vi "TCP_IP Jayasingha Richou Odier.vi"() -> ()   [LabVIEW 2019]
panel:
  out "VIBRATION ANGLE":dynamicdata(graph)
  out "VOL  DB":dynamicdata(graph)
  out "GAZ PPM":dynamicdata(graph)
  out "LUMINOSITE LUX":dynamicdata(graph)
  out "HUMIDITE %":dynamicdata(graph)
  out "TEMPERATURE":dynamicdata(graph)
  out "Nombre de lignes lues":i32
  out "?":dbl
  out "?":dbl
  out "?":dbl
  out "?":dbl
  out "CUMUL DES POINTS":dbl
  out "Oui (vert) / Non (rouge)":bool
  out "Points gaz":dbl
  out "Points Humidité":dbl
  out "Points Temperature":dbl
  out "?":dbl(slide) scale=0.0..0.005
  out "?":dbl(slide) scale=0.0..0.005
  out "?":dbl(slide) scale=0.0..0.005
  out "?":dbl(slide) scale=0.0..0.005
  out "?":dbl(slide) scale=0.0..0.005
  out "?":dbl(slide) scale=0.0..0.005
  out "?":dbl(slide) scale=0.0..0.005
  out "Données de sortie":dbl[][](array[numeric])
  out "Valeur de la  i ème ligne lue":dbl[](array[numeric])
  in  "stop":bool
  # "COUNTER"
  # "HUMIDITÉ"
  # "TEMPERATURE"
  # "LUMINOSITÉ"
  # "GAZ"
  # "VOLUME PIC"
  # "VOLUME AMBIANT"
  # "VIBRATIONS"
  # "A t il le droit d'avoir une compensation ?"
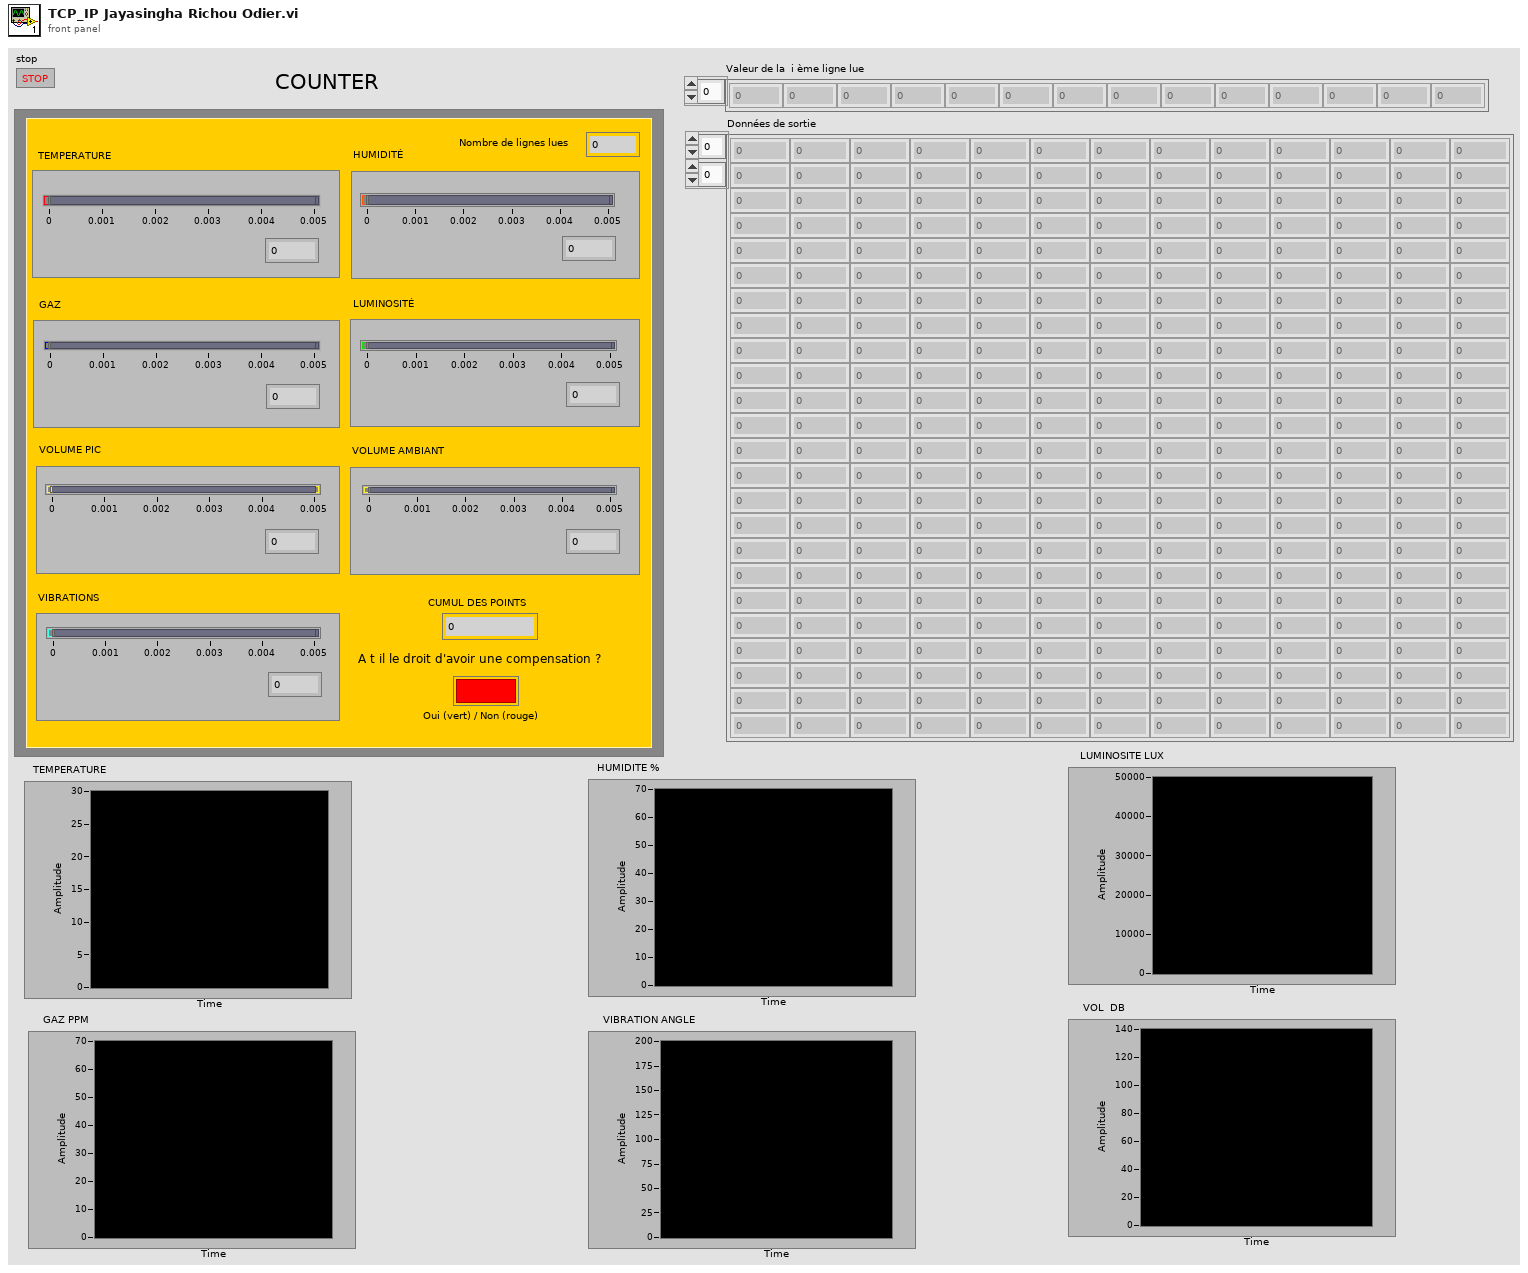
[diagram p1: front panel]
types:
  T1 = enum16{"Standard", "Buffered", "CRLF", "Immediate"}
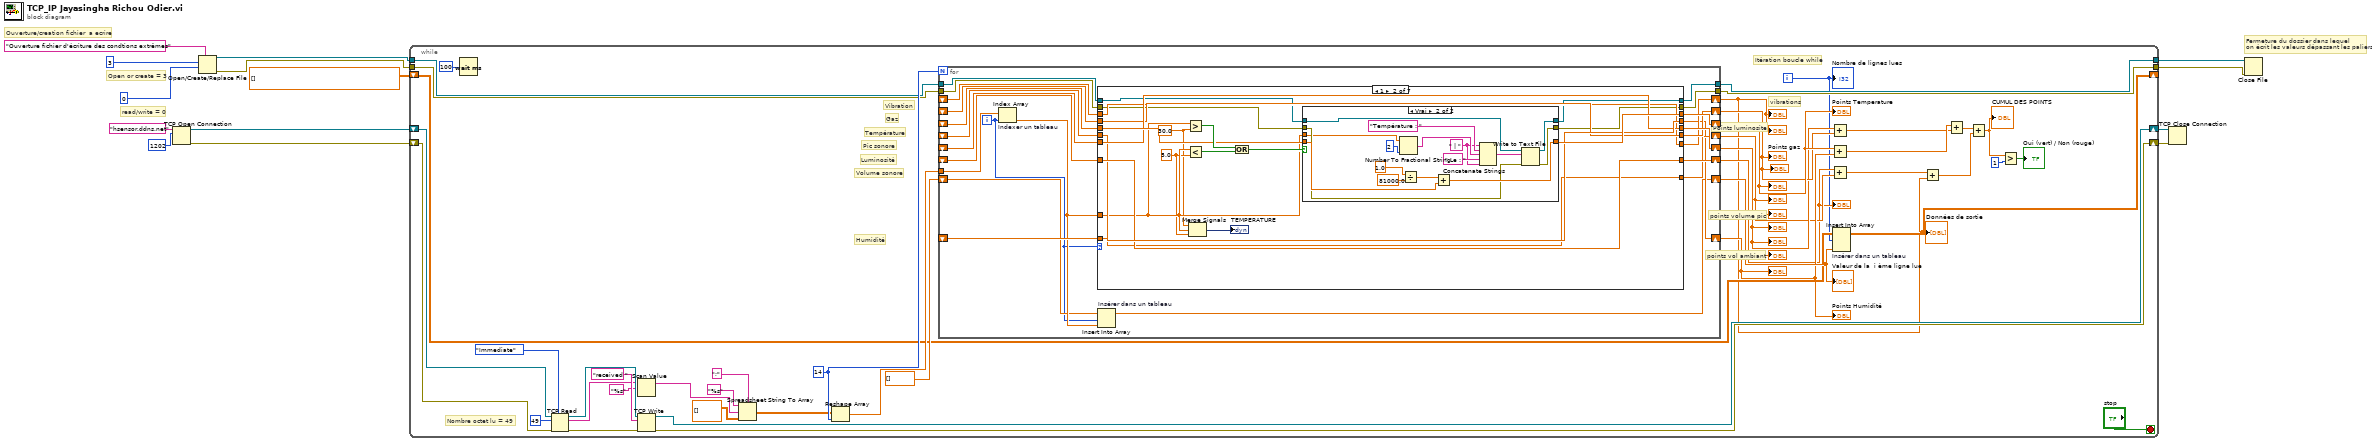
[diagram p0: block diagram]
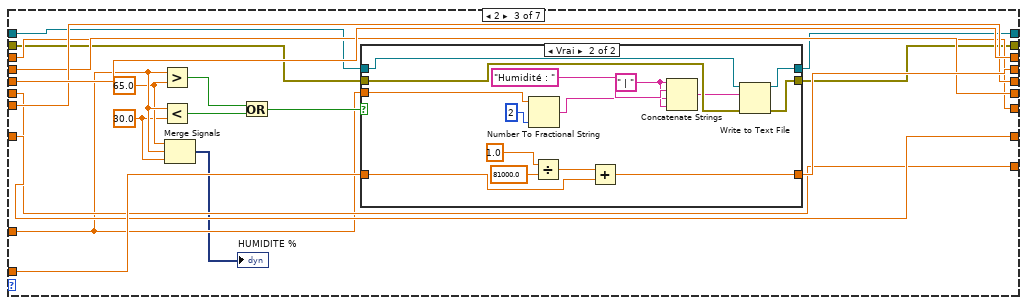
[diagram p4: hidden frame]
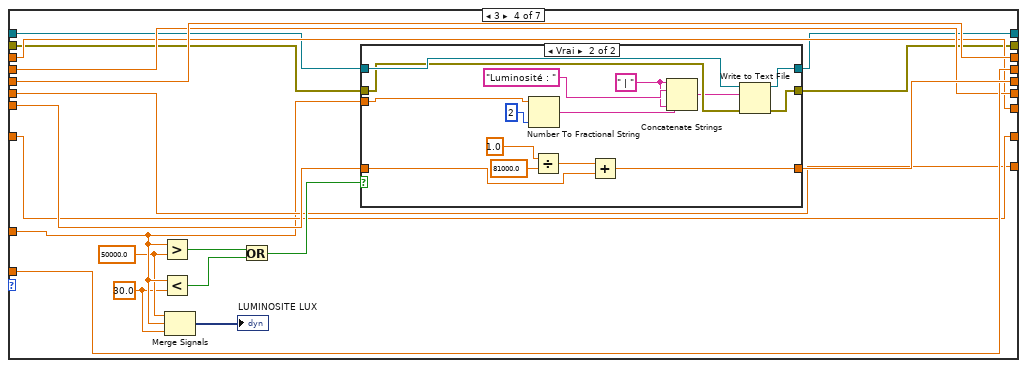
[diagram p6: hidden frame]
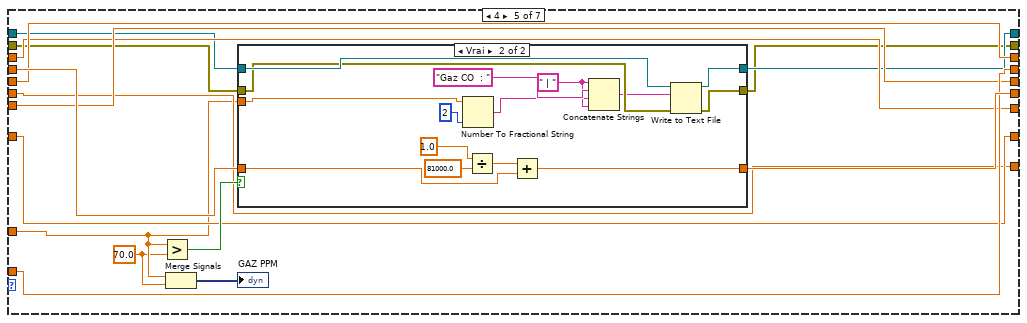
[diagram p8: hidden frame]
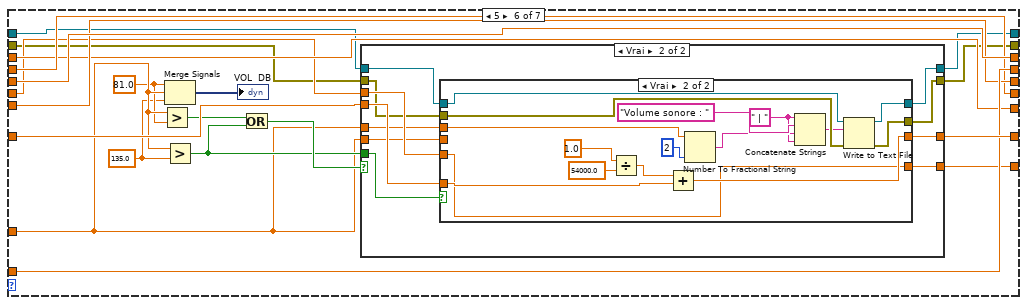
[diagram p10: hidden frame]
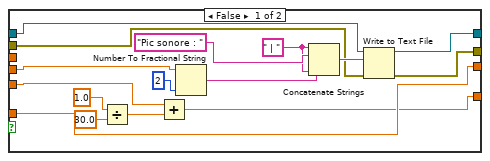
[diagram p12: hidden frame]
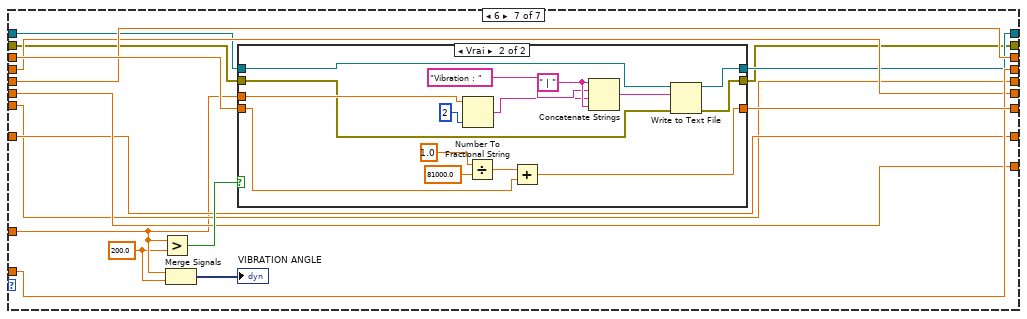
[diagram p13: hidden frame]
diagram:
  # "Fermeture du dossier dans lequel \non écrit les valeurs dépassant les paliers"
  # "read/write = 0"
  # "Open or create = 3"
  # "Ouverture/creation fichier  a ecrire"
  n1 = TCP Open Connection(address="hsensor.ddns.net", remote port or service name=u16 1202) -> (connection ID=w10:refnum<k5>, error out=w9:errorcluster)  [unwired: 3 in]
  n2 = Open/Create/Replace File(prompt="Ouverture fichier d'écriture des condtions extrêmes", operation (0:open)=3, access (0:read/write)=0) -> (refnum out=w3:refnum<file>, error out=w4:errorcluster)  [unwired: 3 in, 1 out]
  n3 = while {
    shift-right: [w57] -> w14
    shift-left: w9 -> [w55]
    shift-right: [w53] -> w11
    shift-left: w10 -> [w52]
    shift-right: [w27] -> _
    shift-left: dbl[][] [] ("array type (2D Dbl)") -> [w29]
    tunnel: w4 -> [w26]
    tunnel: w3 -> [w25]
    tunnel: [w24] -> w2
    tunnel: [w23] -> w1
    i -> [w15]
    stop <- "stop" stop-if-true
    w42 = 14 ("dimension size")
    # "Itération boucle while"
    # "vibrations"
    # "points vol ambiant"
    # "points volume pic"
    # "Points luminosite"
    # "Nombre octet lu = 49"
    # "Vibration"
    # "Pic sonore"
    # "Volume sonore"
    # "Gaz"
    # "Luminosité"
    # "Humidité"
    # "Température"
    n4 = Wait (ms)(milliseconds to wait=u32 100) -> ()  [unwired: 1 out]
    n5 = TCP Read(connection ID=w52, bytes to read=49, error in (no error)=w55, 7:T1."Immediate" ("mode (standard)")) -> (connection ID out=w54:refnum<k5>, data out=w47:string, error out=w58:errorcluster)  [unwired: 1 in]
    n6 = Scan Value(string=w47, format string="%s") -> (output string=w32:string)  [unwired: 1 in, 1 out]
    n7 = TCP Write(connection ID=w54, data in="received " ("data out"), error in (no error)=w58) -> (connection ID out=w53:refnum<k5>, error out=w57:errorcluster)  [unwired: 1 in, 1 out]
    n8 = Spreadsheet String To Array(delimiter (Tab)=";", format string="%s", spreadsheet string=w32, array type (2D Dbl)=dbl[][] []) -> (array=w28:dbl[][])
    n9 = Reshape Array "Reshape Array"(w28, w42) -> (w41:dbl[])
    n10 = for {
      N: w42 -> [_]
      shift-right: [w65] -> w30
      shift-left: dbl[] [] ("array type (2D Dbl)") -> [w66]
      tunnel: w41 -> [w59]
      shift-right: [w81] -> w22
      shift-left: _ -> [w80]
      shift-right: [w69] -> w21
      shift-left: _ -> [w68]
      shift-right: [w78] -> w19
      shift-left: _ -> [w79]
      shift-right: [w76] -> w20
      shift-left: _ -> [w77]
      shift-right: [w74] -> w17
      shift-left: _ -> [w75]
      shift-right: [w72] -> w18
      shift-left: _ -> [w73]
      shift-right: [w71] -> w16
      shift-left: _ -> [w70]
      tunnel: w26 -> [w64]
      tunnel: w25 -> [w63]
      tunnel: [w62] -> w24
      tunnel: [w61] -> w23
      i -> [w60]
      n11 = Index Array "Indexer un tableau"(array=w59, index=w60) -> (element=w67:dbl)
      n12 = case shown="1" w60 {
        tunnel: [w90 w106 w142 w179 w215 w254 w316] -> w81
        tunnel: w80 -> [w90 w105 w142 w179 w215 w254 w316]
        tunnel: [w89 w104 w144 w178 w214 w253 w315] -> w69
        tunnel: w79 -> [w88 w103 w141 w180 w213 w252 w311]
        tunnel: [w88 w103 w141 w181 w213 w252 w311] -> w78
        tunnel: w77 -> [w87 w102 w140 w177 w218 w251 w312]
        tunnel: [w87 w102 w140 w177 w216 w251 w312] -> w76
        tunnel: w75 -> [w86 w101 w139 w176 w212 w256 w313]
        tunnel: [w86 w101 w139 w176 w212 w255 w313] -> w74
        tunnel: w73 -> [w85 w100 w138 w175 w211 w246 w314]
        tunnel: [w85 w100 w138 w175 w211 w245 w314] -> w72
        tunnel: [w84 w99 w137 w174 w210 w250 w318] -> w71
        tunnel: w70 -> [w84 w99 w137 w174 w210 w250 w317]
        tunnel: w68 -> [w89 w104 w143 w178 w214 w253 w315]
        tunnel: w67 -> [_ w94 w132 w169 w205 w240 w306]
        tunnel: w64 -> [w83 w98 w135 w172 w208 w243 w310]
        tunnel: w63 -> [w82 w97 w136 w173 w209 w244 w309]
        tunnel: [w83 w96 w134 w171 w206 w241 w307] -> w62
        tunnel: [w82 w95 w133 w170 w207 w242 w308] -> w61
        frame 0, Default {
        }
        frame 1 {
          w93 = 5.0 ("y")
          w92 = 30.0 ("y")
          n13 = Greater?(x=w94, y=w92) -> (0:w109:bool)
          n14 = Less?(x=w94, y=w93) -> (x < y?=w108:bool)
          n15 = Merge Signals(w92, w94, w93) -> (→"TEMPERATURE":dynamicdata)
          n16 = Or(x=w109, y=w108) -> (x .or. y?=w107:bool)
          n17 = case shown="Vrai" w107 {
            tunnel: [w112 w125] -> w106
            tunnel: w105 -> [w112 w123]
            tunnel: w98 -> [w110 w122]
            tunnel: w97 -> [w111 w121]
            tunnel: [w110 w120] -> w96
            tunnel: [w111 w119] -> w95
            tunnel: w94 -> [_ w113]
            frame False {
            }
            frame True {
              w114 = " | "
              n18 = Number To Fractional String(number=w113, precision (6)=i16 2 ("précision (6)")) -> (F-format string=w117:string)  [unwired: 2 in]
              n19 = Divide(x=1.0, y=81000.0) -> (x/y=w126:dbl)
              n20 = Add(x=w126, y=w123) -> (x+y=w125:dbl)
              n21 = Concatenate Strings(w114, "Température : ", w117, " Le : ", w114) -> (w116:string)
              n22 = Write to Text File(file (use dialog)=w121, text=w116, error in=w122) -> (refnum out=w119:refnum<file>, error out=w120:errorcluster)  [unwired: 1 in, 1 out]
            }
          }
        }
        frame 2 {
          w131 = 65.0 ("y")
          w130 = 30.0 ("y")
          n23 = Greater?(x=w132, y=w131) -> (0:w147:bool)
          n24 = Less?(x=w132, y=w130) -> (x < y?=w146:bool)
          n25 = Merge Signals(w131, w132, w130) -> (→"HUMIDITE %":dynamicdata)
          n26 = Or(x=w147, y=w146) -> (x .or. y?=w145:bool)
          n27 = case shown="Vrai" w145 {
            tunnel: [w150 w162] -> w144
            tunnel: w143 -> [w150 w160]
            tunnel: w136 -> [w149 w159]
            tunnel: w135 -> [w148 w158]
            tunnel: [w148 w157] -> w134
            tunnel: [w149 w156] -> w133
            tunnel: w132 -> [_ w155]
            frame False {
            }
            frame True {
              w153 = " | "
              n28 = Number To Fractional String(number=w155, precision (6)=i16 2 ("précision (6)")) -> (F-format string=w152:string)  [unwired: 2 in]
              n29 = Divide(x=1.0, y=81000.0) -> (x/y=w165:dbl)
              n30 = Add(x=w165, y=w160) -> (x+y=w162:dbl)
              n31 = Concatenate Strings(w153, "Humidité : ", w152, w153) -> (w151:string)
              n32 = Write to Text File(file (use dialog)=w159, text=w151, error in=w158) -> (refnum out=w156:refnum<file>, error out=w157:errorcluster)  [unwired: 1 in, 1 out]
            }
          }
        }
        frame 3 {
          w168 = 50000.0 ("y")
          w167 = 30.0 ("y")
          n33 = Greater?(x=w169, y=w168) -> (0:w183:bool)
          n34 = Less?(x=w169, y=w167) -> (x < y?=w184:bool)
          n35 = Merge Signals(w168, w169, w167) -> (→"LUMINOSITE LUX":dynamicdata)
          n36 = Or(x=w183, y=w184) -> (x .or. y?=w182:bool)
          n37 = case shown="Vrai" w182 {
            tunnel: [w187 w199] -> w181
            tunnel: w180 -> [w187 w197]
            tunnel: w173 -> [w186 w196]
            tunnel: w172 -> [w185 w195]
            tunnel: [w185 w194] -> w171
            tunnel: [w186 w193] -> w170
            tunnel: w169 -> [_ w192]
            frame False {
            }
            frame True {
              w188 = " | "
              n38 = Number To Fractional String(number=w192, precision (6)=i16 2 ("précision (6)")) -> (F-format string=w191:string)  [unwired: 2 in]
              n39 = Divide(x=1.0, y=81000.0) -> (x/y=w200:dbl)
              n40 = Add(x=w200, y=w197) -> (x+y=w199:dbl)
              n41 = Concatenate Strings(w188, "Luminosité : ", w191, w188) -> (w189:string)
              n42 = Write to Text File(file (use dialog)=w196, text=w189, error in=w195) -> (refnum out=w193:refnum<file>, error out=w194:errorcluster)  [unwired: 1 in, 1 out]
            }
          }
        }
        frame 4 {
          w204 = 70.0 ("y")
          n43 = Greater?(x=w205, y=w204) -> (0:w217:bool)
          n44 = Merge Signals(w205, w204) -> (→"GAZ PPM":dynamicdata)
          n45 = case shown="Vrai" w217 {
            tunnel: w218 -> [w221 w231]
            tunnel: [w221 w233] -> w216
            tunnel: w209 -> [w220 w230]
            tunnel: w208 -> [w219 w229]
            tunnel: [w220 w228] -> w207
            tunnel: [w219 w227] -> w206
            tunnel: w205 -> [_ w226]
            frame False {
            }
            frame True {
              w224 = " | "
              n46 = Number To Fractional String(number=w226, precision (6)=i16 2 ("précision (6)")) -> (F-format string=w223:string)  [unwired: 2 in]
              n47 = Divide(x=1.0, y=81000.0) -> (x/y=w234:dbl)
              n48 = Add(x=w234, y=w231) -> (x+y=w233:dbl)
              n49 = Concatenate Strings(w224, "Gaz CO  : ", w223, w224) -> (w222:string)
              n50 = Write to Text File(file (use dialog)=w230, text=w222, error in=w229) -> (refnum out=w228:refnum<file>, error out=w227:errorcluster)  [unwired: 1 in, 1 out]
            }
          }
        }
        frame 5 {
          w238 = 135.0 ("y")
          w239 = 81.0 ("y")
          n51 = Greater?(x=w240, y=w239) -> (0:w248:bool)
          n52 = Merge Signals(w239, w240, w238) -> (→"VOL  DB":dynamicdata)
          n53 = Greater?(x=w240, y=w238) -> (0:w247:bool)
          n54 = Or(x=w248, y=w247) -> (x .or. y?=w249:bool)
          n55 = case shown="Vrai" w249 {
            tunnel: w256 -> [w260 w270]
            tunnel: [w260 w269] -> w255
            tunnel: w247 -> [_ w271]
            tunnel: w246 -> [w259 w268]
            tunnel: [w259 w267] -> w245
            tunnel: w240 -> [_ w266]
            tunnel: w244 -> [w258 w265]
            tunnel: w243 -> [w257 w264]
            tunnel: [w258 w263] -> w242
            tunnel: [w257 w262] -> w241
            tunnel: w240 -> [_ w261]
            frame False {
            }
            frame True {
              n56 = case shown="Vrai" w271 {
                tunnel: w270 -> [w284 w300]
                tunnel: [w284 w299] -> w269
                tunnel: w268 -> [w283 w298]
                tunnel: [w282 w298] -> w267
                tunnel: w266 -> [_ w296]
                tunnel: w265 -> [w276 w295]
                tunnel: w264 -> [w275 w294]
                tunnel: [w273 w293] -> w263
                tunnel: [w274 w292] -> w262
                tunnel: w261 -> [w272 _]
                frame False {
                  w277 = " | "
                  n57 = Divide(x=1.0, y=30.0) -> (x/y=w285:dbl)
                  n58 = Add(x=w283, y=w285) -> (x+y=w282:dbl)
                  n59 = Number To Fractional String(number=w272, precision (6)=i16 2 ("précision (6)")) -> (F-format string=w280:string)  [unwired: 2 in]
                  n60 = Concatenate Strings(w277, "Pic sonore : ", w280, w277) -> (w281:string)
                  n61 = Write to Text File(file (use dialog)=w276, text=w281, error in=w275) -> (refnum out=w273:refnum<file>, error out=w274:errorcluster)  [unwired: 1 in, 1 out]
                }
                frame True {
                  w288 = " | "
                  n62 = Divide(x=1.0, y=54000.0) -> (x/y=w302:dbl)
                  n63 = Add(x=w302, y=w300) -> (x+y=w299:dbl)
                  n64 = Number To Fractional String(number=w296, precision (6)=i16 2 ("précision (6)")) -> (F-format string=w289:string)  [unwired: 2 in]
                  n65 = Concatenate Strings(w288, "Volume sonore : ", w289, w288) -> (w290:string)
                  n66 = Write to Text File(file (use dialog)=w295, text=w290, error in=w294) -> (refnum out=w293:refnum<file>, error out=w292:errorcluster)  [unwired: 1 in, 1 out]
                }
              }
            }
          }
        }
        frame 6 {
          w305 = 200.0 ("y")
          n67 = Greater?(x=w306, y=w305) -> (0:w319:bool)
          n68 = Merge Signals(w306, w305) -> (→"VIBRATION ANGLE":dynamicdata)
          n69 = case shown="Vrai" w319 {
            tunnel: [w322 w334] -> w318
            tunnel: w317 -> [w322 w333]
            tunnel: w306 -> [_ w331]
            tunnel: w310 -> [w320 w330]
            tunnel: w309 -> [w321 w329]
            tunnel: [w321 w328] -> w308
            tunnel: [w320 w327] -> w307
            frame False {
            }
            frame True {
              w326 = " | "
              n70 = Number To Fractional String(number=w331, precision (6)=i16 2 ("précision (6)")) -> (F-format string=w324:string)  [unwired: 2 in]
              n71 = Divide(x=1.0, y=81000.0) -> (x/y=w335:dbl)
              n72 = Add(x=w335, y=w333) -> (x+y=w334:dbl)
              n73 = Concatenate Strings(w326, "Vibration : ", w324, w326) -> (w323:string)
              n74 = Write to Text File(file (use dialog)=w329, text=w323, error in=w330) -> (refnum out=w328:refnum<file>, error out=w327:errorcluster)  [unwired: 1 in, 1 out]
            }
          }
        }
      }
      n75 = Insert Into Array "Insérer dans un tableau"(array=w66, index=w60, new element=w67) -> (w65:dbl[])
    }
    "Points Humidité" <- w21
    "?" <- w19
    "Points gaz" <- w20
    "?" <- w18
    "?" <- w17
    "?" <- w16
    "Valeur de la  i ème ligne lue" <- w30
    "?" <- w22
    "?" <- w20
    "?" <- w18
    "?" <- w16
    "Points Temperature" <- w22
    "?" <- w21
    "?" <- w19
    "?" <- w17
    n76 = Add(x=w19, y=w20) -> (x+y=w38:dbl)
    n77 = Add(x=w22, y=w21) -> (x+y=w39:dbl)
    n78 = Add(x=w17, y=w18) -> (x+y=w40:dbl)
    n79 = Insert Into Array "Insérer dans un tableau"(array=w29, index (row)=w15, new element=w30) -> (w27:dbl[][])  [unwired: 1 in]
    "Données de sortie" <- w27
    n80 = Add(x=w40, y=w16) -> (x+y=w37:dbl)
    n81 = Add(x=w39, y=w38) -> (x+y=w36:dbl)
    n82 = Add(x=w36, y=w37) -> (x+y=w35:dbl)
    "CUMUL DES POINTS" <- w35
    n83 = Greater?(x=w35, y=1) -> (0:→"Oui (vert) / Non (rouge)":bool)
    "Nombre de lignes lues" <- w15
  }
  n84 = TCP Close Connection(connection ID=w11, error in (no error)=w14) -> ()  [unwired: 1 in, 2 out]
  n85 = Close File(refnum=w1, error in=w2) -> ()  [unwired: 2 out]
